vi "Read Points.vi"(8 "error in (no error)":errorcluster, 11 "FSM.Edge in":refnum<class "FSM.Edge.lvclass">) -> (0 "error out":errorcluster, 2 "Points":cluster{"x":i16, "y":i16}[](array[cluster]), 3 "FSM.Edge out":refnum<class "FSM.Edge.lvclass">)   [LabVIEW 2020, in "FSM.Edge.lvclass"]
uses:
  FSM.Edge.lvclass
  FSM.Edge.lvclass/FSM.Edge.ctl
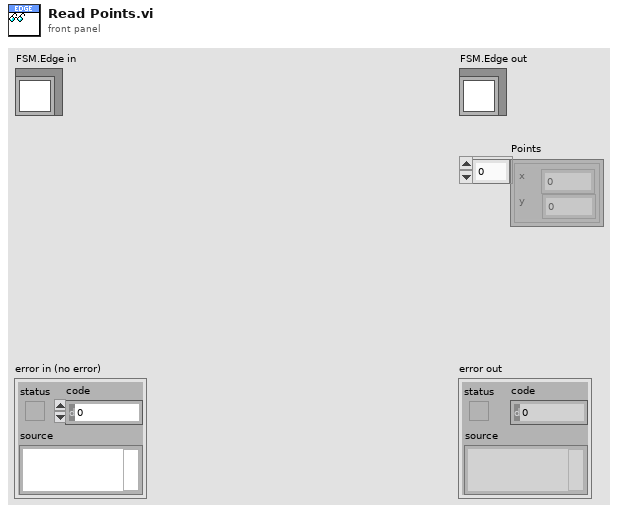
[diagram p1: front panel]
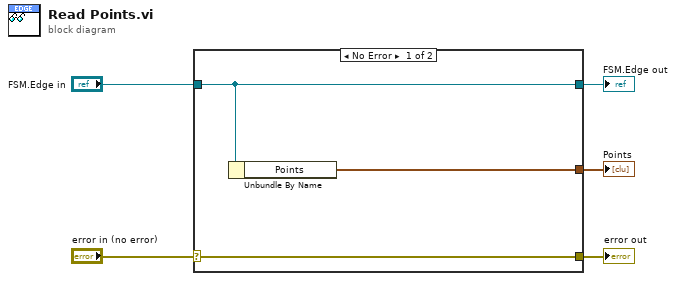
[diagram p0: block diagram]
diagram:
  n1 = case shown="No Error" "error in (no error)" {
    selector: "error in (no error)" -> [w8 w9]
    tunnel: [w8 w9] -> w4
    tunnel: [w7 w10] -> w2
    tunnel: "FSM.Edge in" -> [w7 w10]
    tunnel: [w6 _] -> w1
    frame No Error {
      n2 = Unbundle By Name(w7) -> ("Points"=w6:cluster{"x":i16, "y":i16}[])
    }
    frame Error {
    }
  }
  "error out" <- w4
  "FSM.Edge out" <- w2
  "Points" <- w1
